vi "setUp.vi"(8 "error in (no error)":errorcluster, 11 "reference in":refnum<class "Test TCP Nested-Caller Two Last Acks.lvclass">) -> (0 "error out":errorcluster, 3 "reference out":refnum<class "Test TCP Nested-Caller Two Last Acks.lvclass">)   [LabVIEW 2020, in "Test TCP Nested-Caller Two Last Acks.lvclass"]
doc: "setUp runs prior to the test method during test execution. Use this method to initialize any object data required by your tests."
uses:
  Test TCP Nested-Caller Two Last Acks.lvclass
  <vilib>/addons/_JKI Toolkits/VI Tester/TestCase.llb/TestCase.lvclass
  <vilib>/ActorFramework/Actor/Actor.lvclass
  <vilib>/ActorFramework/Message Queue/Message Queue.lvclass
  Source/Protocols/TCP Strategy/TCP Stream Listener/TCP Stream Listener.lvclass
  Source/Protocols/TCP Strategy/TCP Stream Initiator/TCP Stream Initiator.lvclass
  Source/Protocols/TCP Strategy/TCP Stream/TCP Stream.lvclass
  Source/Ciphers/AES/AES.lvclass
  Source/Ciphers/AES/Ton Plomp Encryption/AES-Modes.ctl
  Source/Ciphers/AES/Ton Plomp Encryption/Encryption.lvlib
  Source/Nested Endpoint/Nested Endpoint/Nested Endpoint.lvclass
  Source/Network Endpoint/Network Endpoint/Network Endpoint.lvclass
  Source/Caller Endpoint/Caller Endpoint/Caller Endpoint.lvclass
  Support/Caller Test Harness/Caller Test Harness/Caller Test Harness.lvclass
  Source/Abstract Classes/Message Stream/Message Stream.lvclass
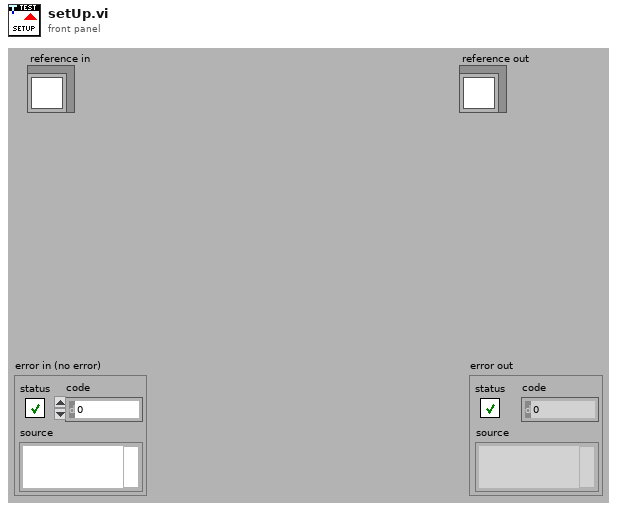
[diagram p1: front panel]
types:
  T1 = typedef "Encryption.lvlib/AES-Modes.ctl" = enum16{"ECB", "CBC", "CFB128", "OFB"}
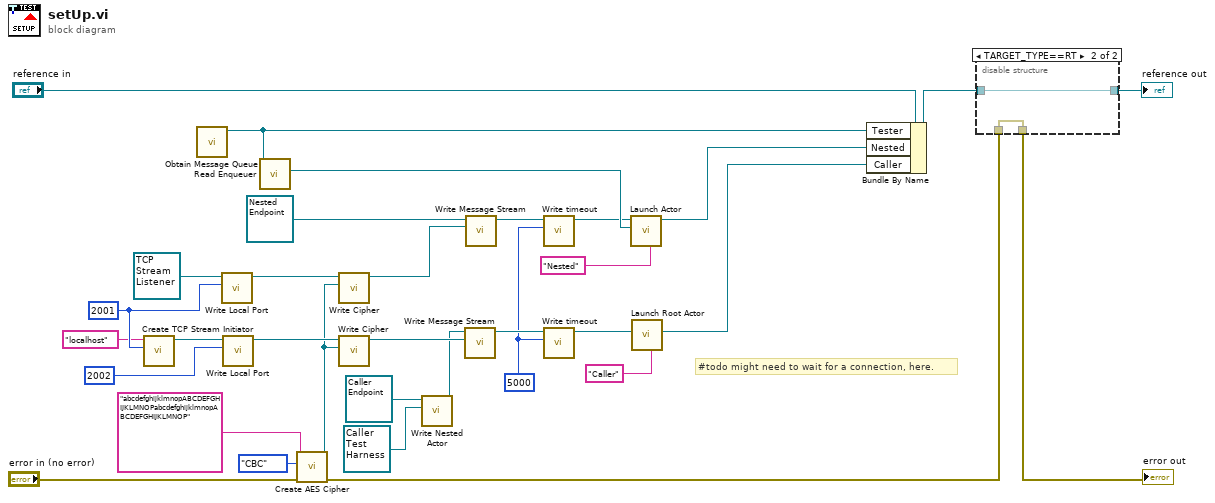
[diagram p0: block diagram]
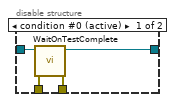
[diagram p2: hidden frame]
diagram:
  w6 = 5000 ("timeout")
  w26 = u16 2001 ("Port")
  # "#todo might need to wait for a connection, here."
  n1 = call "Create TCP Stream Initiator.vi"("Remote Port"=w26, "Remote Address"="localhost" ("IP Address")) -> ("TCP Stream Initiator"=w28:refnum<class "TCP Stream Initiator.lvclass">)  [unwired: 9 in]
  n2 = call <vilib>:"Obtain Message Queue.vi"() -> ("Message Queue"=w12:refnum<class "Message Queue.lvclass">)  [unwired: 10 in, 1 out]
  n3 = call "Write Local Port.vi"("local port"=w26, "TCP Stream in"=refnum<class "TCP Stream Listener.lvclass"> refnum ("TCP Stream Listener.lvclass")) -> ("TCP Stream out"=w25:refnum<class "TCP Stream Listener.lvclass">)  [unwired: 9 in]
  n4 = call "Write Local Port.vi"("local port"=u16 2002, "TCP Stream in"=w28) -> ("TCP Stream out"=w24:refnum<class "TCP Stream Initiator.lvclass">)  [unwired: 9 in]
  n5 = call <vilib>:"Read Enqueuer.vi"("Message Queue"=w12) -> ("Message Enqueuer"=w29:refnum<class "Message Enqueuer.lvclass">)  [unwired: 10 in]
  n6 = call "Create AES Cipher.vi"("error in (no error)"="error in (no error)", "Operation Mode"=AES-Modes."CBC", "Cipher Key"="abcdefghijklmnopABCDEFGHIJKLMNOPabcdefghijklmnopABCDEFGHIJKLMNOP") -> ("error out"=w20:errorcluster, "AES out"=w19:refnum<class "AES.lvclass">)  [unwired: 7 in]
  n7 = call "Write Cipher.vi"("Cipher"=w19, "Message Stream in"=w25) -> ("Message Stream out"=w17:refnum<class "TCP Stream Listener.lvclass">)  [unwired: 9 in]
  n8 = call "Write Cipher.vi"("Cipher"=w19, "Message Stream in"=w24) -> ("Message Stream out"=w16:refnum<class "TCP Stream Initiator.lvclass">)  [unwired: 9 in]
  n9 = call "Write Nested Actor.vi"("Nested Actor"=refnum<class "Caller Test Harness.lvclass"> refnum ("Caller Test Harness.lvlib:Caller Test Harness.lvclass"), "Caller Endpoint in"=refnum<class "Caller Endpoint.lvclass"> refnum ("Caller Endpoint.lvlib:Caller Endpoint.lvclass")) -> ("Caller Endpoint out"=w2:refnum<class "Caller Endpoint.lvclass">)  [unwired: 9 in]
  n10 = call "Write Message Stream.vi"("Message Stream"=w16, "Network Endpoint in"=w2) -> ("Network Endpoint out"=w8:refnum<class "Caller Endpoint.lvclass">)  [unwired: 9 in]
  n11 = call "Write Message Stream.vi"("Message Stream"=w17, "Network Endpoint in"=refnum<class "Nested Endpoint.lvclass"> refnum ("Nested Endpoint.lvlib:Nested Endpoint.lvclass")) -> ("Network Endpoint out"=w10:refnum<class "Nested Endpoint.lvclass">)  [unwired: 9 in]
  n12 = call "Write timeout.vi"("timeout"=w6, "Network Endpoint in"=w10) -> ("Network Endpoint out"=w9:refnum<class "Nested Endpoint.lvclass">)  [unwired: 9 in]
  n13 = call "Write timeout.vi"("timeout"=w6, "Network Endpoint in"=w8) -> ("Network Endpoint out"=w7:refnum<class "Caller Endpoint.lvclass">)  [unwired: 9 in]
  n14 = call <vilib>:"Launch Actor.vi"("Debug Alias"="Nested", "Actor-to-Caller Enqueuer"=w29, "Actor"=w9) -> ("Caller-To-Actor Enqueuer"=w14:refnum<class "Message Enqueuer.lvclass">)  [unwired: 7 in, 1 out]
  n15 = call <vilib>:"Launch Root Actor.vi"("Debug Alias"="Caller", "Actor"=w7) -> ("Actor's Enqueuer"=w13:refnum<class "Message Enqueuer.lvclass">)  [unwired: 8 in, 1 out]
  n16 = Bundle By Name(cluster="reference in", "Tester"=w12, "Nested"=w14, "Caller"=w13) -> (w30:refnum<class "Test TCP Nested-Caller Two Last Acks.lvclass">)
  n17 = disable-structure shown="TARGET_TYPE==RT" {
    disable-tunnel: w20 -> [w37 w38]
    disable-tunnel: [w36 w38] -> w33
    disable-tunnel: [w35 w39] -> w31
    disable-tunnel: w30 -> [w34 w39]
    frame condition #0 (active) {
      n18 = call <vilib>:"WaitOnTestComplete.vi"("error in (no error)"=w37, "TestCase in"=w34) -> ("error out"=w36:errorcluster, "TestCase out"=w35:refnum<class "Test TCP Nested-Caller Two Last Acks.lvclass">)  [unwired: 8 in]
    }
    frame condition #1 {
    }
  }
  "error out" <- w33
  "reference out" <- w31
